vi "Position Controller_student.vi"(4 "I":dbl, 6 "P":dbl=1.0, 9 "Y Error":dbl, 10 "X Error":dbl, 11 "Next Waypoint":i32[](array[numeric])) -> (1 "Controller_Outer":dbl, 2 "Controller_Inner":dbl)   [LabVIEW 2012]
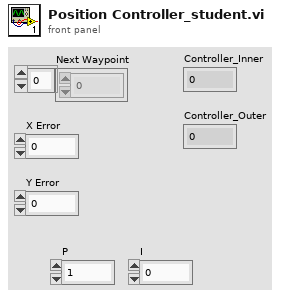
[diagram p1: front panel]
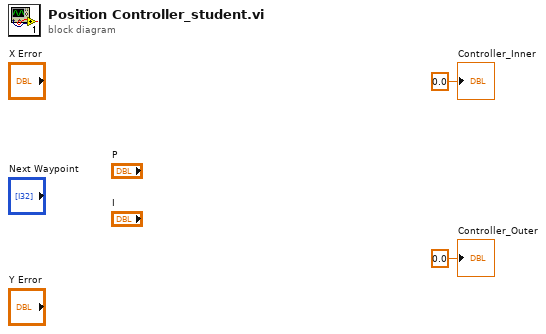
[diagram p0: block diagram]
diagram:
  "Controller_Outer" <- 0.0 ("Controller_Outer")
  "Controller_Inner" <- 0.0 ("Controller_Inner")
